vi "Watermark.vi"(0 "Watermark IN":T1={"Show? (F)"=TRUE, "Type"=enum."Image", "Opacity (%)"=10.0, "Rotate(°)"=0.0, "Position"={"Position"=enum."Center (text section)", "X"=0.0, "Y"=0.0}, "Image path"=path "", "Scaled(%)"=100.0, "Image refnum"=refnum, "Text"="CONFIDENTIAL", "Font"={"Name"="", "Size"=-1.0, "Color"=0}, "Font refnum"=refnum, "Alignment"=enum."Center", "Automatic"=FALSE}, 7 "pageNum":i32=1, 11 "error in (no error)":errorcluster, 13 "Page dimensions":T6={"Start at page"=1, "Page Size"=0, "Orientation"=enum."Landscape", "widht"=792.0, "height"=72.0, "Margin left"=72.0, "Margin right"=72.0, "Margin top"=72.0, "Margin bottom"=72.0, "X0"=0.0, "X1"=612.0, "Y0"=0.0, "Y1"=792.0} {"Page Size" items=["Custom", "LETTER", "NOTE", "LEGAL", "TABLOID", "EXECUTIVE", "POSTCARD", "A0", "A1", "A2", "A3", "A4", "A5", "A6", "A7", "A8", "A9", "A10", "B0", "B1", "B2", "B3", "B4", "B5", "B6", "B7", "B8", "B9", "B10", "ARCH_E", "ARCH_D", "ARCH_C", "ARCH_B", "ARCH_A", "FLSA", "FLSE", "HALFLETTER", "_11X17", "ID_1", "ID_2", "ID_3", "LEDGER", "CROWN_QUARTO", "LARGE_CROWN_QUARTO", "DEMY_QUARTO", "ROYAL_QUARTO", "CROWN_OCTAVO", "LARGE_CROWN_OCTAVO", "DEMY_OCTAVO", "ROYAL_OCTAVO", "SMALL_PAPERBACK", "PENGUIN_SMALL_PAPERBACK", "PENGUIN_LARGE_PAPERBACK"]}) -> (4 "Watermark OUT":T1={"Show? (F)"=TRUE, "Type"=enum."Image", "Opacity (%)"=10.0, "Rotate(°)"=0.0, "Position"={"Position"=enum."Center (text section)", "X"=0.0, "Y"=0.0}, "Image path"=path "", "Scaled(%)"=100.0, "Image refnum"=refnum, "Text"="CONFIDENTIAL", "Font"={"Name"="", "Size"=-1.0, "Color"=0}, "Font refnum"=refnum, "Alignment"=enum."Center", "Automatic"=FALSE}, 15 "error out":errorcluster)   [LabVIEW 2019]
doc: "Version 1.0\nDeveloped by Jean-Marc Simard\nCopyright © 2010, Exaprom Inc.\nAll rights reserved.\nLicense: BSD\n\nWith iTextSharp 4.1.6 (http://itextsharp.sourceforge.net)\nunder Mozilla Public License Version 1.1\n(http://www.mozilla.org/MPL/MPL-1.1.html)"
uses:
  <userlib>/Exaprom PDF/Controls/Page Controls/Page dimensions.ctl
  <userlib>/Exaprom PDF/Controls/Page Controls/Page size.ctl
  <userlib>/Exaprom PDF/Controls/Page Controls/Page Orientation.ctl
  <userlib>/Exaprom PDF/Controls/Header, Footer and Watermark Controls/Watermark cluster2.ctl
  <userlib>/Exaprom PDF/Controls/Header, Footer and Watermark Controls/Watermark Position.ctl
  C:/Program Files/National Instruments/LabVIEW 2019/user.lib/Exaprom PDF/DLL/itextsharp.dll
  DLL/itextsharp.dll
  <userlib>/Exaprom PDF/Controls/Font Controls/Font size.ctl
  <userlib>/Exaprom PDF/Controls/Font Controls/Font color.ctl
  <userlib>/Exaprom PDF/Controls/Header, Footer and Watermark Controls/Header footer horiz alignment.ctl
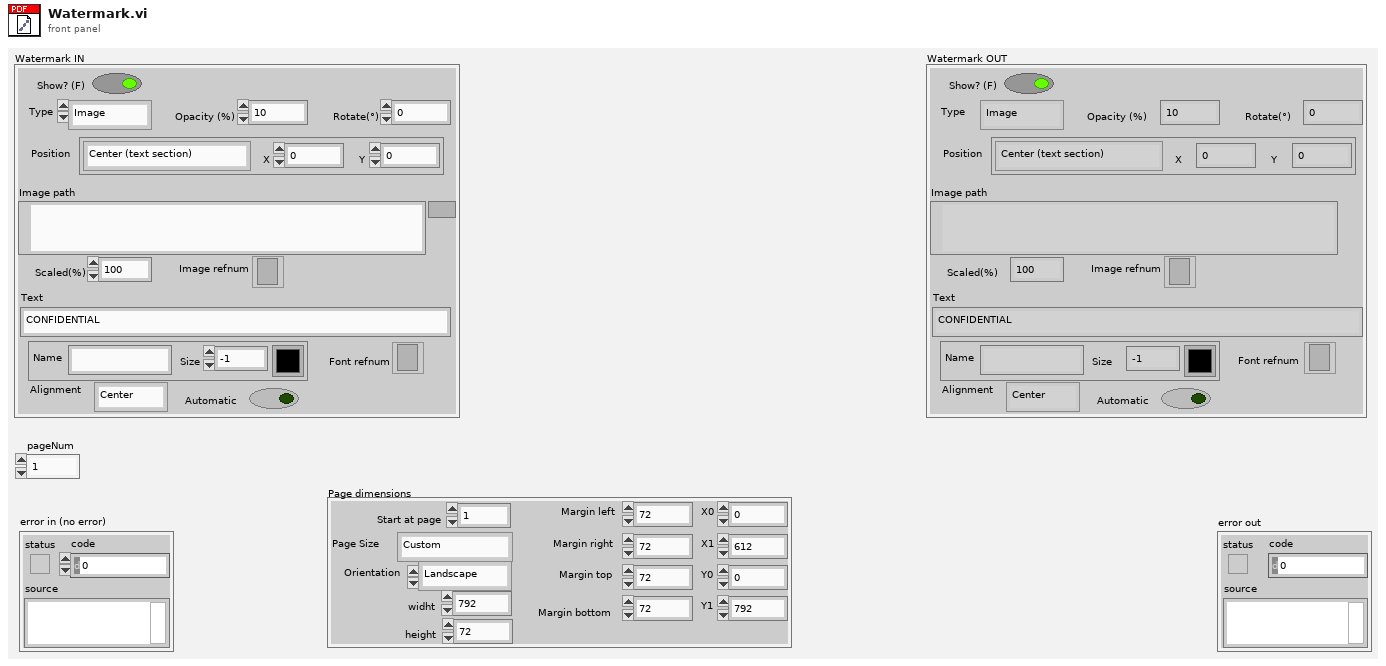
[diagram p1: front panel]
types:
  T1 = typedef "Watermark cluster2.ctl" = cluster{"Show? (F)":bool, "Type":enum16{"Image", "Text"}, "Opacity (%)":sgl, "Rotate(°)":sgl, "Position":cluster{"Position":T2, "X":sgl, "Y":sgl}, "Image path":path, "Scaled(%)":sgl, "Image refnum":refnum<k24>, "Text":string, "Font":cluster{"Name":string, "Size":T3, "Color":T4}, "Font refnum":refnum<k24>, "Alignment":T5, "Automatic":bool}
  T2 = typedef "Watermark Position.ctl" = enum16{"Absolute", "Center (page)", "Center (text section)"}
  T3 = typedef "Font size.ctl" = sgl
  T4 = typedef "Font color.ctl" = u32
  T5 = typedef "Header footer horiz alignment.ctl" = enum16{"Left", "Center", "Right"}
  T6 = typedef "Page dimensions.ctl" = cluster{"Start at page":i32, "Page Size":T7, "Orientation":T8, "widht":sgl, "height":sgl, "Margin left":sgl, "Margin right":sgl, "Margin top":sgl, "Margin bottom":sgl, "X0":sgl, "X1":sgl, "Y0":sgl, "Y1":sgl}
  T7 = typedef "Page size.ctl" = i32
  T8 = typedef "Page Orientation.ctl" = enum16{"Portrait", "Landscape"}
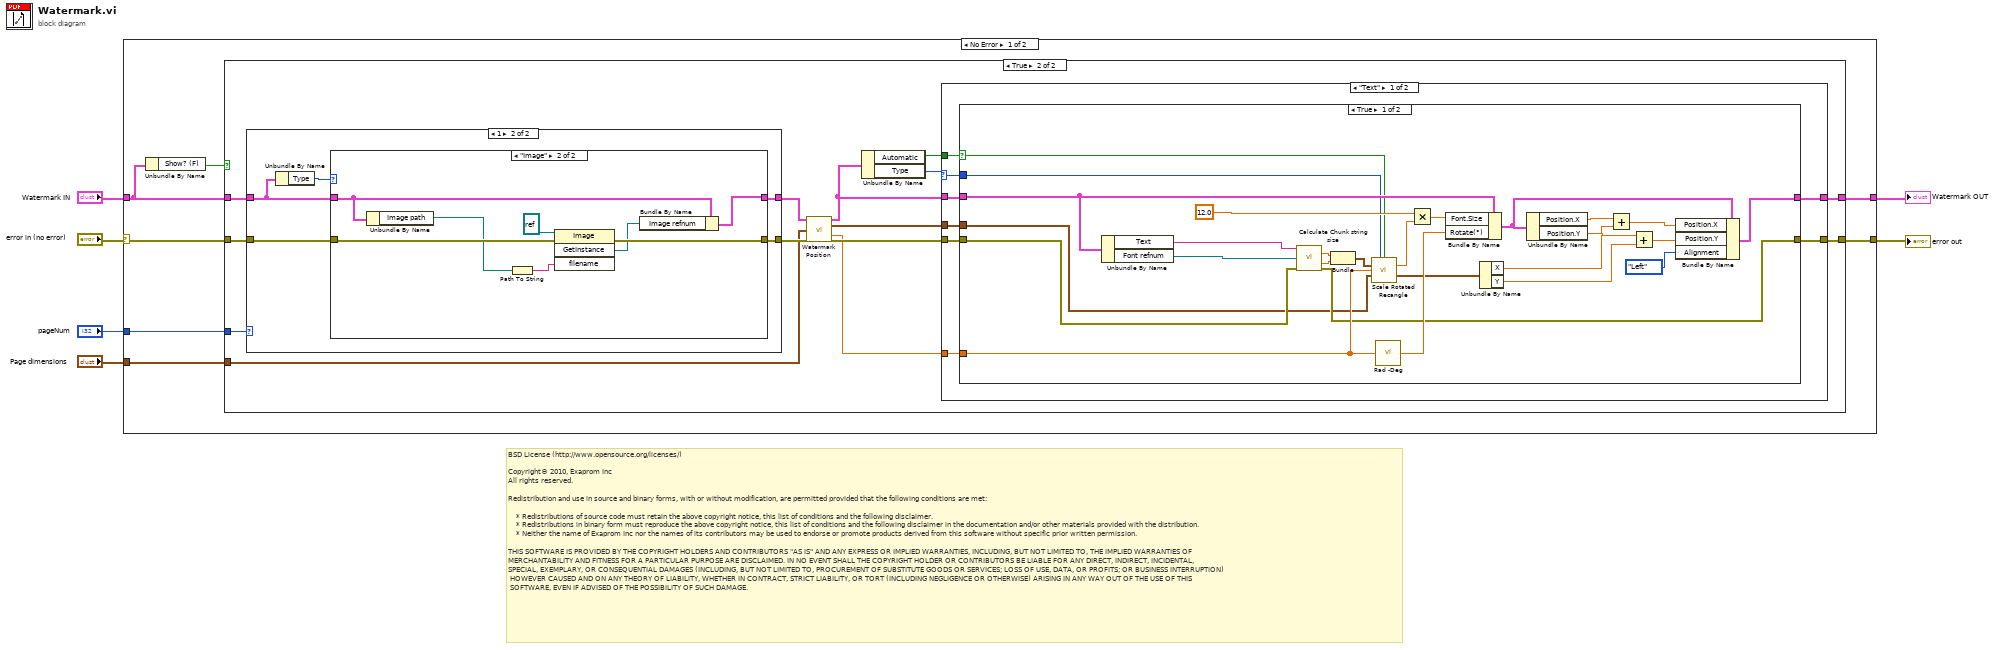
[diagram p0: block diagram]
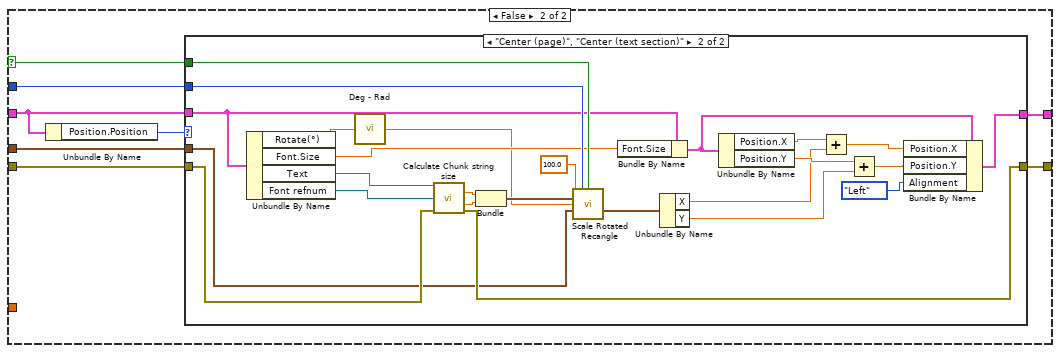
[diagram p3: hidden frame]
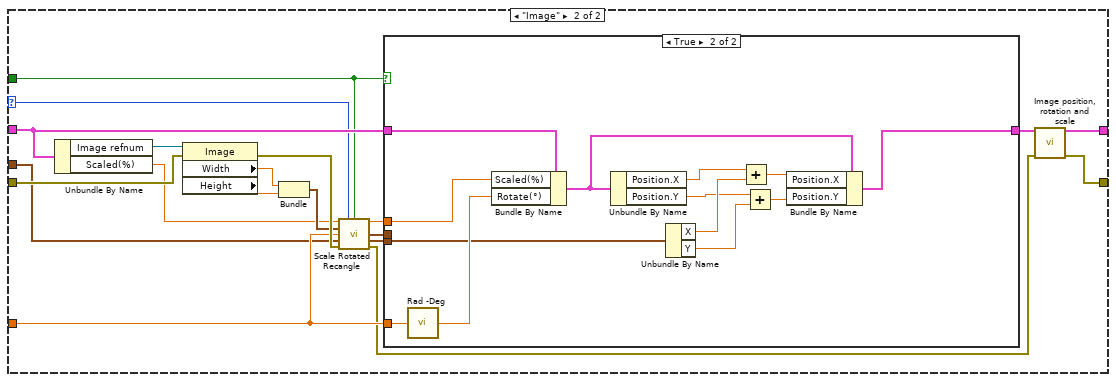
[diagram p5: hidden frame]
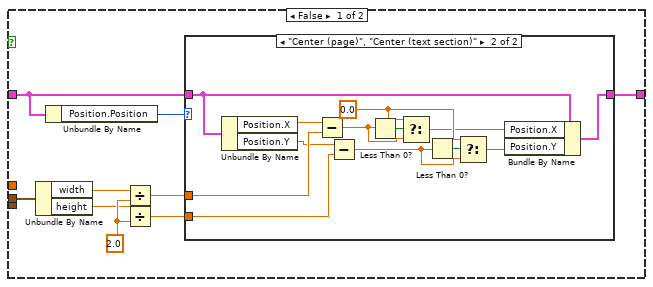
[diagram p6: hidden frame]
diagram:
  # "BSD License (http://www.opensource.org/licenses/)\n\nCopyright© 2010, Exaprom Inc\nAll rights reserved.\n\nRedistribution and use in source and binary forms, with or without modification, are permitted provided that the following conditions are met:\n\n    * Redistributions of source code must retain the above copyright notice, this list of conditions and the following disclaimer.\n    * Redistributions in binary form must reproduce the above copyright notice, this list of conditions and the following disclaimer in the documentation and/or other materials provided with the distribution.\n    * Neither the name of Exaprom Inc nor the names of its contributors may be used to endorse or promote products derived from this software without specific prior written permission.\n\nTHIS SOFTWARE IS PROVIDED BY THE COPYRIGHT HOLDERS AND CONTRIBUTORS \"AS IS\" AND ANY EXPRESS OR IMPLIED WARRANTIES, INCLUDING, BUT NOT LIMITED TO, THE IMPLIED WARRANTIES OF \nMERCHANTABILITY AND FITNESS FOR A PARTICULAR PURPOSE ARE DISCLAIMED. IN NO EVENT SHALL THE COPYRIGHT HOLDER OR CONTRIBUTORS BE LIABLE FOR ANY DIRECT, INDIRECT, INCIDENTAL,\nSPECIAL, EXEMPLARY, OR CONSEQUENTIAL DAMAGES (INCLUDING, BUT NOT LIMITED TO, PROCUREMENT OF SUBSTITUTE GOODS OR SERVICES; LOSS OF USE, DATA, OR PROFITS; OR BUSINESS INTERRUPTION)\n HOWEVER CAUSED AND ON ANY THEORY OF LIABILITY, WHETHER IN CONTRACT, STRICT LIABILITY, OR TORT (INCLUDING NEGLIGENCE OR OTHERWISE) ARISING IN ANY WAY OUT OF THE USE OF THIS\n SOFTWARE, EVEN IF ADVISED OF THE POSSIBILITY OF SUCH DAMAGE."
  n1 = case shown="No Error" "error in (no error)" {
    selector: "error in (no error)" -> [w10 w172]
    tunnel: "Watermark IN" -> [w8 w171]
    tunnel: "pageNum" -> [w9 _]
    tunnel: "Page dimensions" -> [w13 _]
    tunnel: [w12 w172] -> w3
    tunnel: [w11 w171] -> w1
    frame No Error {
      n2 = Unbundle By Name(w8) -> ("Show? (F)"=w7:bool)
      n3 = case shown="True" w7 {
        tunnel: w8 -> [w15 w29]
        tunnel: w13 -> [_ w21]
        tunnel: [w14 w20] -> w12
        tunnel: [w15 w19] -> w11
        tunnel: w10 -> [w14 w18]
        tunnel: w9 -> [_ w16]
        frame False {
        }
        frame True {
          n4 = case shown="1" w16 {
            tunnel: w18 -> [w154 w160]
            tunnel: w29 -> [w155 w159]
            tunnel: [w154 w157] -> w24
            tunnel: [w155 w156] -> w25
            frame 0, Default {
            }
            frame 1 {
              n5 = Unbundle By Name(w159) -> ("Type"=w158:enum16{"Image", "Text"})
              n6 = case shown="\"Image\"" w158 {
                tunnel: w159 -> [w162 w170]
                tunnel: w160 -> [w161 w164]
                tunnel: [w162 w169] -> w156
                tunnel: [w161 w168] -> w157
                frame "Text", Default {
                }
                frame "Image" {
                  n7 = Unbundle By Name(w170) -> ("Image path"=w163:path)
                  n8 = Path To String(path=w163) -> (string=w166:string)
                  n9 = invoke class="Image" method="GetInstance"(reference=refnum<k24> refnum ("image"), error in=w164, "filename"=w166) -> (error out=w168:errorcluster, "GetInstance"=w165:refnum<k24>)  [unwired: 1 in, 2 out]
                  n10 = Bundle By Name(cluster=w170, "Image refnum"=w165) -> (w169:T1)
                }
              }
            }
          }
          n11 = call <userlib>:"Watermark Position.vi"("Watermark Cluster IN"=w25, "Page dimensions"=w21, "error in (no error)"=w24) -> ("Watermark Cluster OUT"=w26:T1, "Box"=w17:cluster{"width":sgl, "height":sgl}, "Angle (rad)"=w23:dbl, "error out"=w27:errorcluster)  [unwired: 9 out]
          n12 = Unbundle By Name(w26) -> ("Automatic"=w22:bool, "Type"=w28:enum16{"Image", "Text"})
          n13 = case shown="\"Text\"" w28 {
            selector: w28 -> [w32 w103]
            tunnel: w27 -> [w30 w109]
            tunnel: w26 -> [w37 w116]
            tunnel: w23 -> [w36 w108]
            tunnel: w22 -> [w34 w102]
            tunnel: [w31 w115] -> w20
            tunnel: [w35 w114] -> w19
            tunnel: w17 -> [w33 w104]
            frame "Text" {
              n14 = case shown="True" w34 {
                selector: w34 -> [w46 w66]
                tunnel: w37 -> [w52 w65]
                tunnel: w36 -> [w57 _]
                tunnel: [w60 w71] -> w35
                tunnel: w33 -> [w48 w68]
                tunnel: w32 -> [w47 w67]
                tunnel: w30 -> [w50 w70]
                tunnel: [w49 w69] -> w31
                frame True {
                  n15 = Unbundle By Name(w52) -> ("Text"=w51:string, "Font refnum"=w38:refnum<k24>)
                  n16 = call <userlib>:"Calculate Chunk string size.vi"("String"=w51, "Font refnum"=w38, "error in (no error)"=w50) -> ("Width"=w54:sgl, "Height"=w55:sgl, "error out"=w49:errorcluster)  [unwired: 2 in, 8 out]
                  n17 = Bundle("Width"=w54, "Height"=w55) -> (w62:cluster{"Width":sgl, "Height":sgl})  [unwired: 1 out]
                  n18 = call <userlib>:"Scale Rotated Recangle.vi"("Type"=w47, "Automatic"=w46, "Original Rectangle"=w62, "Angle (rad)"=w57, "Page or text zone size"=w48) -> ("Scale Factor"=w58:dbl, "Offset"=w61:cluster{"X":dbl, "Y":dbl})  [unwired: 2 in, 7 out]
                  n19 = call <userlib>:"Rad -Deg.vi"("Radians iN"=w57) -> ("Degrees out"=w63:dbl)
                  n20 = Multiply(x=T3 12.0 ("Font.Size"), y=w58) -> (x*y=w56:dbl)
                  n21 = Bundle By Name(cluster=w52, "Font.Size"=w56, "Rotate(°)"=w63) -> (w45:T1)
                  n22 = Unbundle By Name(w61) -> ("X"=w40:dbl, "Y"=w39:dbl)
                  n23 = Unbundle By Name(w45) -> ("Position.X"=w44:sgl, "Position.Y"=w43:sgl)
                  n24 = Add(x=w44, y=w40) -> (x+y=w42:dbl)
                  n25 = Add(x=w43, y=w39) -> (x+y=w41:dbl)
                  n26 = Bundle By Name(cluster=w45, "Position.X"=w42, "Position.Y"=w41, "Alignment"=Header_footer_horiz_alignment."Left") -> (w60:T1)
                }
                frame False {
                  n27 = Unbundle By Name(w65) -> ("Position.Position"=w64:T2)
                  n28 = case shown="\"Center (page)\", \"Center (text section)\"" w64 {
                    tunnel: [w73 w96] -> w71
                    tunnel: w70 -> [w72 w91]
                    tunnel: [w72 w90] -> w69
                    tunnel: w68 -> [_ w89]
                    tunnel: w67 -> [_ w88]
                    tunnel: w66 -> [_ w87]
                    tunnel: w65 -> [w73 w79]
                    frame "Absolute", Default {
                    }
                    frame "Center (page)", "Center (text section)" {
                      n29 = Unbundle By Name(w79) -> ("Rotate(°)"=w76:sgl, "Font.Size"=w77:T3, "Text"=w92:string, "Font refnum"=w74:refnum<k24>)
                      n30 = call <userlib>:"Deg - Rad.vi"("Degrees IN"=w76) -> ("Radian OUT"=w75:dbl)
                      n31 = call <userlib>:"Calculate Chunk string size.vi"("String"=w92, "Font refnum"=w74, "error in (no error)"=w91) -> ("Width"=w93:sgl, "Height"=w94:sgl, "error out"=w90:errorcluster)  [unwired: 2 in, 8 out]
                      n32 = Bundle("Width"=w93, "Height"=w94) -> (w98:cluster{"Width":sgl, "Height":sgl})  [unwired: 1 out]
                      n33 = call <userlib>:"Scale Rotated Recangle.vi"("Scaled(%)"=sgl 100.0, "Type"=w88, "Automatic"=w87, "Original Rectangle"=w98, "Angle (rad)"=w75, "Page or text zone size"=w89) -> ("Offset"=w97:cluster{"X":dbl, "Y":dbl})  [unwired: 1 in, 8 out]
                      n34 = Bundle By Name(cluster=w79, "Font.Size"=w77) -> (w86:T1)
                      n35 = Unbundle By Name(w97) -> ("X"=w81:dbl, "Y"=w80:dbl)
                      n36 = Unbundle By Name(w86) -> ("Position.X"=w85:sgl, "Position.Y"=w84:sgl)
                      n37 = Add(x=w85, y=w81) -> (x+y=w83:dbl)
                      n38 = Add(x=w84, y=w80) -> (x+y=w82:dbl)
                      n39 = Bundle By Name(cluster=w86, "Position.X"=w83, "Position.Y"=w82, "Alignment"=Header_footer_horiz_alignment."Left") -> (w96:T1)
                    }
                  }
                }
              }
            }
            frame "Image" {
              n40 = Unbundle By Name(w116) -> ("Image refnum"=w110:refnum<k24>, "Scaled(%)"=w100:sgl)
              n41 = property class="Image"(reference=w110, error in=w109) -> (error out=w117:errorcluster, "Width"=w111:sgl, "Height"=w112:sgl)  [unwired: 1 out]
              n42 = Bundle("Width"=w111, "Height"=w112) -> (w101:cluster{"Width":sgl, "Height":sgl})  [unwired: 1 out]
              n43 = call <userlib>:"Scale Rotated Recangle.vi"("Scaled(%)"=w100, "Type"=w103, "Automatic"=w102, "Original Rectangle"=w101, "Angle (rad)"=w108, "Page or text zone size"=w104, "error in (no error)"=w117) -> ("Scale Factor (%)"=w107:dbl, "Scaled Rectangle"=w105:cluster{"width":dbl, "height":dbl}, "Offset"=w106:cluster{"X":dbl, "Y":dbl}, "error out"=w99:errorcluster)  [unwired: 5 out]
              n44 = case shown="True" w102 {
                tunnel: w116 -> [w124 w152]
                tunnel: w108 -> [_ w151]
                tunnel: [w121 w149] -> w113
                tunnel: w107 -> [_ w142]
                tunnel: w106 -> [_ w141]
                tunnel: w105 -> [w120 _]
                frame False {
                  w126 = sgl 2.0 ("ScaledHeight")
                  n45 = Unbundle By Name(w120) -> ("width"=w119:dbl, "height"=w118:dbl)
                  n46 = Unbundle By Name(w124) -> ("Position.Position"=w125:T2)
                  n47 = Divide(x=w119, y=w126) -> (x/y=w123:dbl)
                  n48 = Divide(x=w118, y=w126) -> (x/y=w122:dbl)
                  n49 = case shown="\"Center (page)\", \"Center (text section)\"" w125 {
                    tunnel: w124 -> [w127 w140]
                    tunnel: [w127 w139] -> w121
                    tunnel: w123 -> [_ w137]
                    tunnel: w122 -> [_ w135]
                    frame "Absolute", Default {
                    }
                    frame "Center (page)", "Center (text section)" {
                      w129 = sgl 0.0 ("t")
                      n50 = Unbundle By Name(w140) -> ("Position.X"=w138:sgl, "Position.Y"=w136:sgl)
                      n51 = Subtract(x=w138, y=w137) -> (x-y=w133:dbl)
                      n52 = Subtract(x=w136, y=w135) -> (x-y=w130:dbl)
                      n53 = Less Than 0?(x=w133) -> (x < 0?=w134:bool)
                      n54 = Select(t=w129, s=w134, f=w133) -> (s? t:f=w128:dbl)
                      n55 = Less Than 0?(x=w130) -> (x < 0?=w132:bool)
                      n56 = Select(t=w129, s=w132, f=w130) -> (s? t:f=w131:dbl)
                      n57 = Bundle By Name(cluster=w140, "Position.X"=w128, "Position.Y"=w131) -> (w139:T1)
                    }
                  }
                }
                frame True {
                  n58 = call <userlib>:"Rad -Deg.vi"("Radians iN"=w151) -> ("Degrees out"=w153:dbl)
                  n59 = Bundle By Name(cluster=w152, "Scaled(%)"=w142, "Rotate(°)"=w153) -> (w150:T1)
                  n60 = Unbundle By Name(w150) -> ("Position.X"=w146:sgl, "Position.Y"=w144:sgl)
                  n61 = Unbundle By Name(w141) -> ("X"=w145:dbl, "Y"=w143:dbl)
                  n62 = Add(x=w146, y=w145) -> (x+y=w148:dbl)
                  n63 = Add(x=w144, y=w143) -> (x+y=w147:dbl)
                  n64 = Bundle By Name(cluster=w150, "Position.X"=w148, "Position.Y"=w147) -> (w149:T1)
                }
              }
              n65 = call <userlib>:"Image position, rotation and scale.vi"("Watermark cluster IN"=w113, "error in (no error)"=w99) -> ("Watermark cluster OUT"=w114:T1, "error out"=w115:errorcluster)  [unwired: 12 out]
            }
          }
        }
      }
    }
    frame Error {
    }
  }
  "error out" <- w3
  "Watermark OUT" <- w1
